vi "AAA Emrax 228 2.0 KLEIN BEELD.vi"() -> ()   [LabVIEW 2020]
doc: "This is a practical example of CAN_READ.\nOn the left hand side of the BD is a disabled code section. One can enable this to log CAN data.\nThe potput of this disabled code segment is the error cluster.\nThan the selected channel will be initiatlized.\nOnce the initialisation is OK a timed while loop will be executed until CAN_READ will signal an error.\nInside of the while loop is the CAN_READ function.\nBuilding up an array of CAN mesages and timestamps is done while this loop executes.\nOnly the last message witch is naturaly empty, because the receive queue is empty, will be ignored.\nThe result is an array of received CAN messages."
uses:
  <instrlib>/KDI Digital Instrumentation/API_for_PCAN_BASIC_FD/TPCANParameter.ctl
  <vilib>/Platform/TimedLoop/XDataNode/XDataNode.xnode
  <vilib>/Platform/TimedLoop/XDataNode/nitl_modes.ctl
  <vilib>/Platform/TimedLoop/XDataNode/XDNodeRunTimeDep.lvlib
  <vilib>/Platform/TimedLoop/XDataNode/wakeup.ctl
  <vilib>/Platform/TimedLoop/XDataNode/timing_clust.ctl
  <instrlib>/KDI Digital Instrumentation/API_for_PCAN_BASIC_FD/TPCANHandle.ctl
  <instrlib>/KDI Digital Instrumentation/API_for_PCAN_BASIC_FD/TPCANBaudrate.ctl
  <instrlib>/Gantner Instruments/Ethernet/Gantner-Instruments HighSpeedPort.llb/e.gate Protocol Type.ctl
  <vilib>/Instr/_visa.llb/VISA Configure Serial Port (Instr).vi
  <vilib>/Utility/file.llb/Write Delimited Spreadsheet (string).vi
  <instrlib>/KDI Digital Instrumentation/API_for_PCAN_BASIC_FD/PCAN Get CHANNEL CONDITION.vi
  <instrlib>/KDI Digital Instrumentation/API_for_PCAN_BASIC_FD/TPCANTimestampFD.ctl
panel:
  out "DC Current":dbl(knob) scale=0.0..140.0
  out "Array 2":u8[][](array[numeric])
  out "Max. Cell Voltage":dbl
  out "DC Voltage":dbl(knob) scale=80.0..120.0
  out "Array":u8[][](array[numeric])
  in  "?":bool
  out "error out 3":errorcluster
  out "error out":errorcluster
  out "Value":dbl[](graph)
  out "Brake pot Input":u32
  out "Torque Shudder":u32
  out "Motor Temp":u32(slide) scale=0.0..100.0
  out "Inverter Temp":u32(slide) scale=0.0..100.0
  out "Modulation":u32
  out "Motor Voltage Magnitude":u32
  out "Flux weakening regulator":u32
  out "RPM Feedback":u32(knob) scale=0.0..6000.0
  out "?":u32(knob) scale=0.0..60.0
  out "?":u32(knob) scale=0.0..60.0
  out "Torque Command":u32
  out "Torque Feedback":u32
  out "Potmeter Input":u32
  out "Elapsed Time":u32
  out "return count":u32
  out "Humidity (%)":string
  out "Pressure (Pa)":string
  out "Temperature (°C)":string
  out "Elapsed Time 2":string
  out "?":dbl[](array[slide]) scale=0.0..1000.0
  out "Temperature 2":dbl[](array[slide]) caption="Thermocouple 1" scale=20.0..50.0
  out "error out 2":errorcluster
  out "Min. Cell Voltage":dbl
  out "x/y":dbl(graph)
  out "Battery Temperature":u8(slide) scale=0.0..50.0
  out "State of Charge":dbl(slide) scale=0.0..100.0
  out "appended array":u8[][](array[numeric])
  out "CAN Timestamp":T1[](array[typedef]) format="%016x"
  # "Emrax 228  -  Motor control"
  # "Atmospheric\nConditions"
  # "Temperatures"
  # "Battery Data"
  # "Power Supply"
  # "Torque"
  # "DC Voltage"
  # "Thrust"
  # "DC Current"
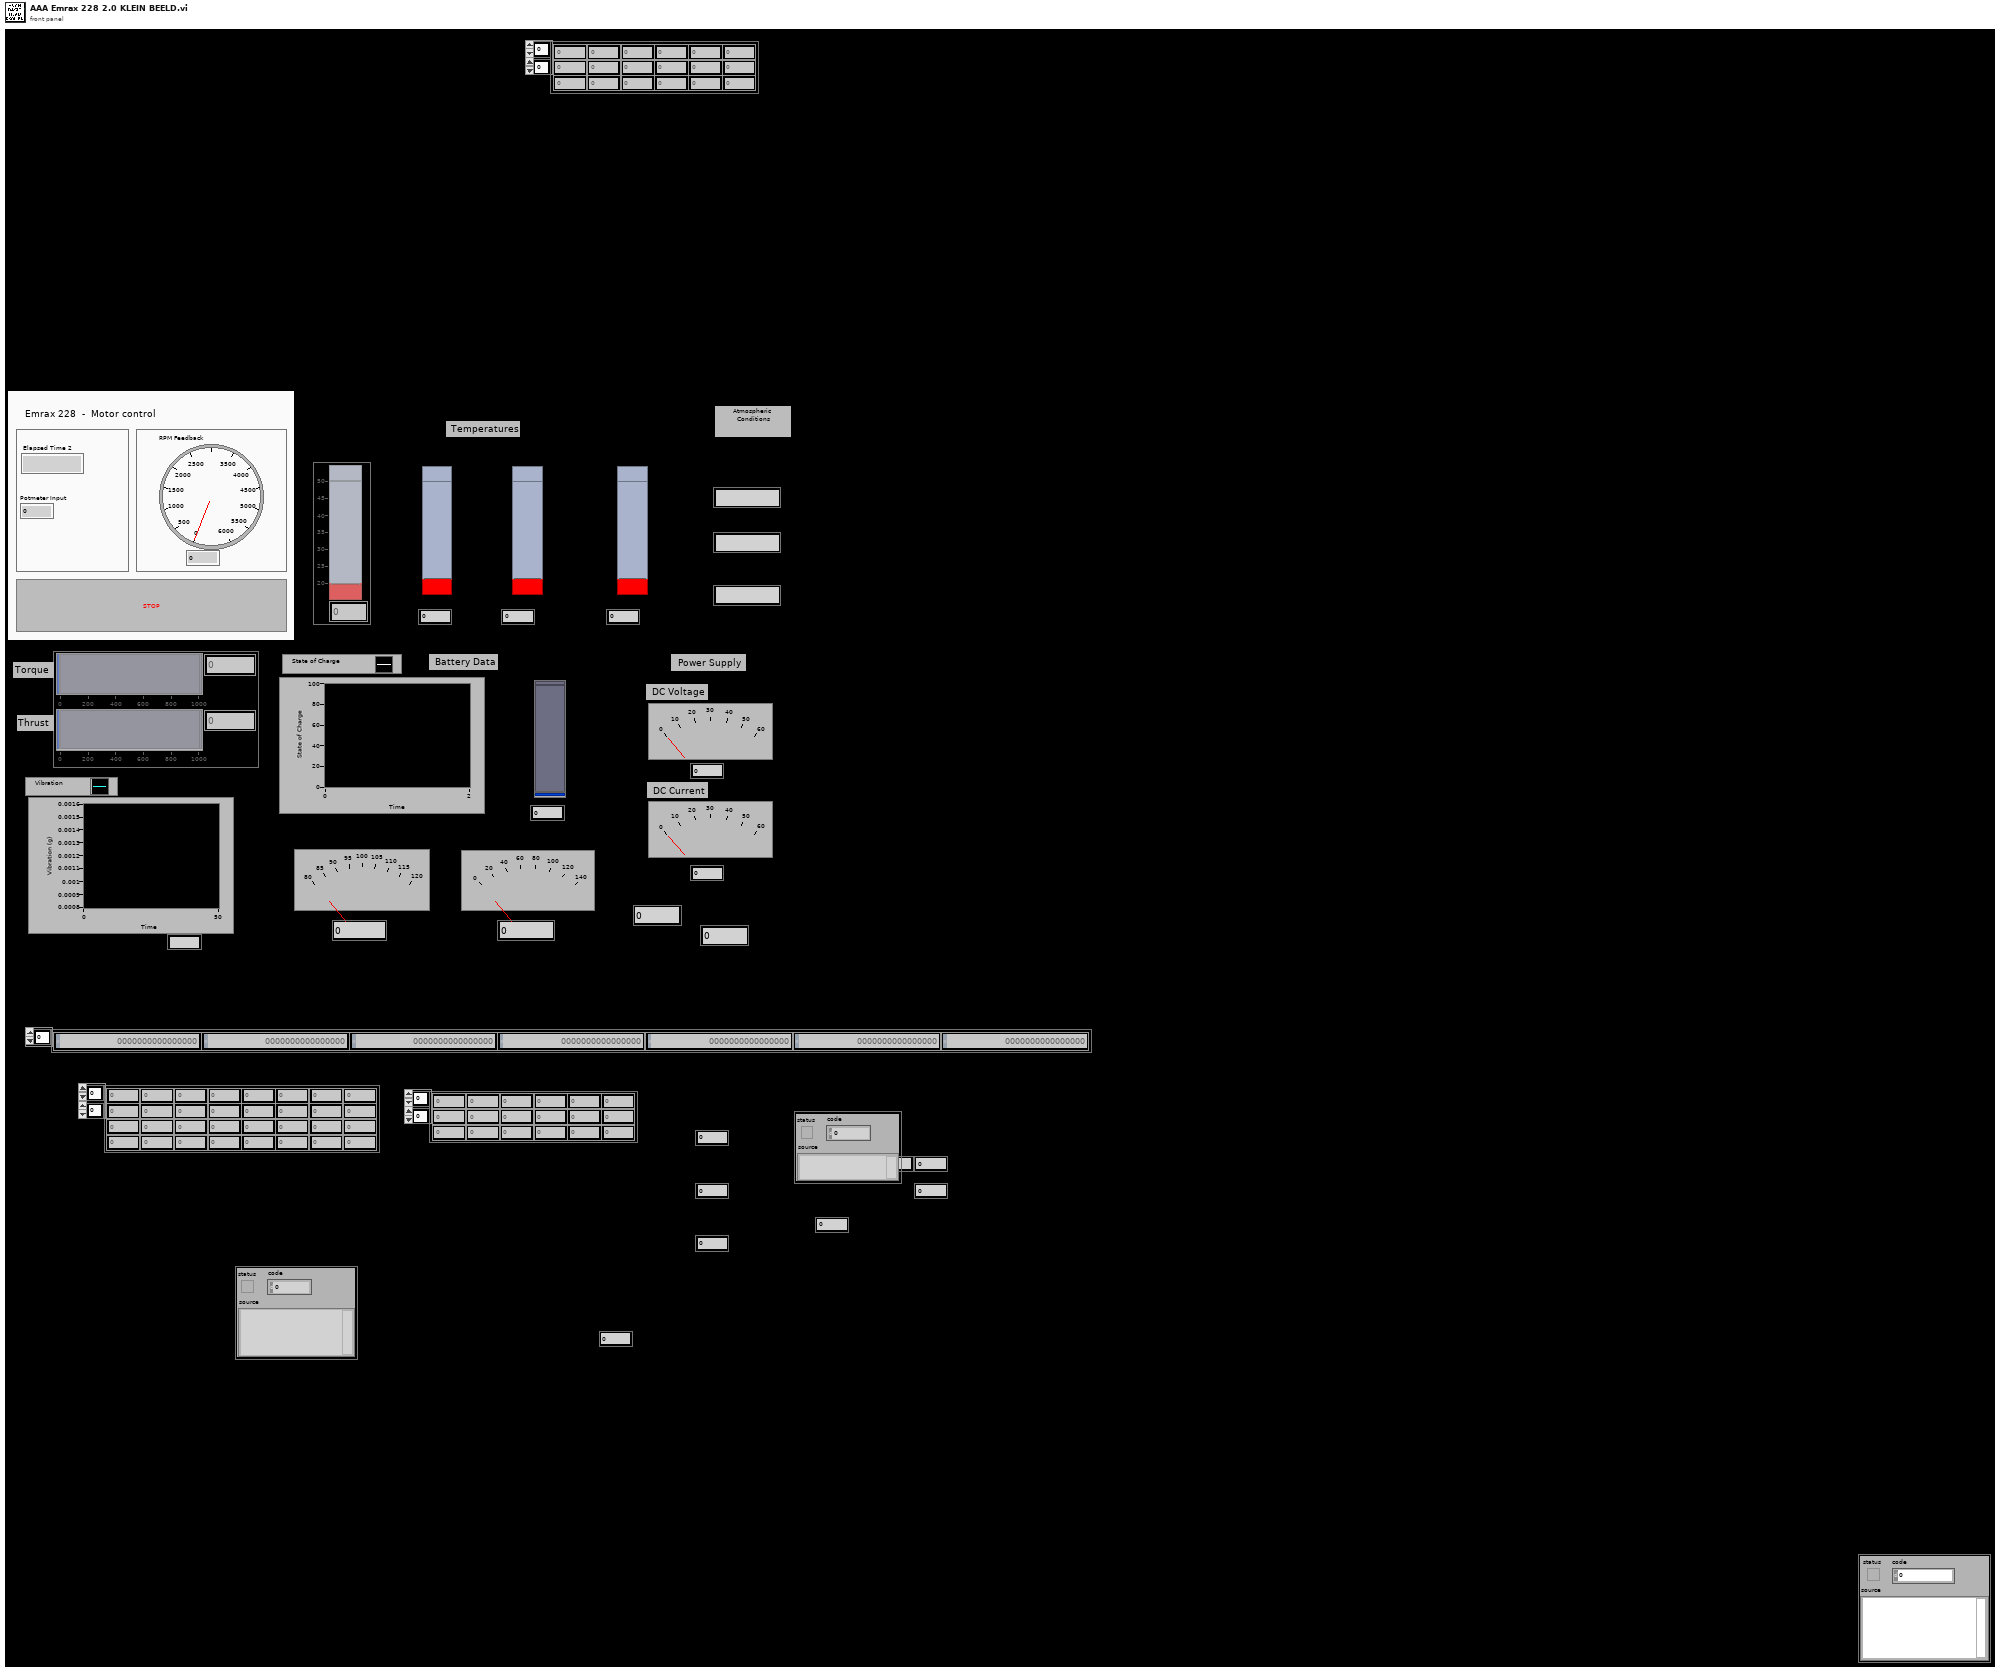
[diagram p1: front panel]
types:
  T1 = typedef "TPCANTimestampFD.ctl" = u64
  T2 = typedef "e.gate Protocol Type.ctl" = enum16{"ASCII", "HighspeedPort Online", "HighspeedPort Buffer (giutility.DLL) ", "PostProcessBuffer (giutility.DLL)", "HighspeedPort Online (giutility.DLL)", "Decode UDBF File (giutility.DLL)"}
  T3 = typedef "TPCANBaudrate.ctl" = enum16{"PCAN_BAUD_1M 0x0014", "PCAN_BAUD_800K 0x0016", "PCAN_BAUD_500K 0x001C", "PCAN_BAUD_250K 0x011C", "PCAN_BAUD_125K 0x031C", "PCAN_BAUD_100K 0x432F", "PCAN_BAUD_95K 0xC34E", "PCAN_BAUD_83K 0x852B", "PCAN_BAUD_50K 0x472F", "PCAN_BAUD_47K 0x1414", "PCAN_BAUD_33K 0x8B2F", "PCAN_BAUD_20K 0x532F", "PCAN_BAUD_10K 0x672F", "PCAN_BAUD_5K 0x7F7F", "User Baudrate"}
  T4 = typedef "TPCANHandle.ctl" = enum16{"PCAN_NONEBUS  0x000", "PCAN_ISABUS1  0x21", "PCAN_ISABUS2  0x22", "PCAN_ISABUS3  0x23", "PCAN_ISABUS4  0x24", "PCAN_ISABUS5  0x25", "PCAN_ISABUS6  0x26", "PCAN_ISABUS7  0x27", "PCAN_ISABUS8  0x28", "PCAN_DNGBUS1  0x31", "PCAN_PCIBUS1  0x41", "PCAN_PCIBUS1  0x42", "PCAN_PCIBUS1  0x43", "PCAN_PCIBUS1  0x44", "PCAN_PCIBUS1  0x45", "PCAN_PCIBUS1  0x46", "PCAN_PCIBUS1  0x47", "PCAN_PCIBUS1  0x48", "PCAN_PCIBUS1  0x409", "PCAN_PCIBUS1  0x40A", "PCAN_PCIBUS1  0x40B", "PCAN_PCIBUS1  0x40C", "PCAN_PCIBUS1  0x40D", "PCAN_PCIBUS1  0x40E", "PCAN_PCIBUS1  0x40F", "PCAN_PCIBUS1  0x410", "PCAN_USBBUS1  0x51", "PCAN_USBBUS2  0x52", "PCAN_USBBUS3  0x53", "PCAN_USBBUS4  0x54", "PCAN_USBBUS5  0x55", "PCAN_USBBUS6  0x56", "PCAN_USBBUS7  0x57", "PCAN_USBBUS8  0x58", "PCAN_USBBUS9  0x509", "PCAN_USBBUS10  0x50A", "PCAN_USBBUS11  0x50B", "PCAN_USBBUS12  0x50C", "PCAN_USBBUS13  0x50D", "PCAN_USBBUS14  0x50E", "PCAN_USBBUS15  0x50F", "PCAN_USBBUS16  0x510", "PCAN_PCCBUS1  0x61", "PCAN_PCCBUS2  0x62", "PCAN_LANBUS1  0x801", "PCAN_LANBUS2  0x802", "PCAN_LANBUS3  0x803", "PCAN_LANBUS4  0x804", "PCAN_LANBUS5  0x805", "PCAN_LANBUS6  0x806", "PCAN_LANBUS7  0x807", "PCAN_LANBUS8  0x808", "PCAN_LANBUS9  0x809", "PCAN_LANBUS10  0x80A", "PCAN_LANBUS11  0x80B", "PCAN_LANBUS12  0x80C", "PCAN_LANBUS13  0x80D", "PCAN_LANBUS14  0x80E", "PCAN_LANBUS15  0x80F", "PCAN_LANBUS16  0x810"}
  T5 = typedef "TPCANParameter.ctl" = enum8{"Not Available", "PCAN device number", "PCAN 5-volt power", "PCAN receive event", "PCAN message filter", "PCAN API version", "PCAN channel version", "PCAN busoff autoreset", "PCAN listen-only", "PCAN log location", "PCAN log status", "PCAN log configure", "PCAN log text", "PCAN channel condition", "PCAN hardware name", "PCAN_RECEIVE_STATUS", "PCAN_CONTROLLER_NUMBER", "PCAN_TRACE_LOCATION ", "PCAN_TRACE_STATUS", "PCAN_TRACE_SIZE", "PCAN_TRACE_CONFIGURE", "PCAN_CHANNEL_IDENTIFYING", "PCAN_CHANNEL_FEATURES", "PCAN_SPEED_ADAPTING", "PCAN_BITRATE_INFO", "PCAN_BITRATE_INFO_FD", "PCAN_BUSSPEED_NOMINAL", "PCAN_BUSSPEED_DATA", "PCAN_IP_ADDRESS", "PCAN_LAN_SERVICE_STATUS", "PCAN_ALLOW_STATUS_FRAMES", "PCAN_ALLOW_RTR_FRAMES", "PCAN_ALLOW_ERROR_FRAMES", "PCAN_INTERFRAME_DELAY", "PCAN_ACCEPTANCE_FILTER_11BIT", "PCAN_ACCEPTANCE_FILTER_29BIT", "PCAN_IO_DIGITAL_CONFIGURATION", "PCAN_IO_DIGITAL_VALUE", "PCAN_IO_DIGITAL_SET", "PCAN_IO_DIGITAL_CLEAR", "PCAN_IO_ANALOG_VALUE"}
  T6 = typedef "Channel Availability.ctl" = enum16{"PCAN_CHANNEL_UNAVAILABLE", "PCAN_CHANNEL_AVAILABLE", "PCAN_CHANNEL_OCCUPIED"}
  T7 = typedef "e.gate Configuration.ctl" = cluster{"connection ID":refnum<k5>, "IPAddress":string, "BufferIndex":i32, "StateMessage":string, "StateCode":i8, "HeaderSize":i32, "BufferSize":i32, "IsBigEndian":i32, "Version":i32, "ChannelCount":i32, "FrameLength":i32, "StartTime":dbl, "dActTimeToSecondFactor":dbl, "StartTimeToDayFactor":dbl, "BufferFillRate":dbl, "SampleRate":dbl, "ChannelData":T8[], "DecodeTimeFormat":string, "SummaryPath":string, "WithCheckSum":i32, "dActTimeDataType":T9, "MaxWriteCount":i32, "MaxReadCount":i32, "TempOffsetRead":i32, "TempLengthRead":i32, "Protocol":T2, "IsSupported":i32, "InputAccessList":i32[], "OutputAccessList":i32[], "DataSource":enum16{"CircleBuffer", "test.con Logger", "test.con Archive"}, "Modules":T10[], "DLL-Handle":T11}
  T8 = typedef "e.gate Channel Data.ctl" = cluster{"VariableName":string, "DataDirection":string, "DataType":string, "DataTypeIndex":T9, "Precision":i16, "FieldLengtht":i16, "ByteCount":i32, "Format":string, "Unit":string, "InputAccessOffset":i32, "OutputAccessOffset":i16, "InputAccessIndex":i16, "OutputAccessIndex":i16, "VarType":string}
  T9 = typedef "e.gate Data Type.ctl" = enum16{"NO", "BOOL", "SINT8", "USINT8", "SINT16", "USINT16", "SINT32", "USINT32", "FLOAT", "SET8", "SET16", "SET32", "DOUBLE", "SINT64", "USINT64", "SET64"}
  T10 = typedef "e.gate Module  Data.ctl" = cluster{"Type":string, "Location":string, "VariablesCount":i16, "UartIndex":i16, "Address":i16, "SystemOffset":i16}
  T11 = typedef "e.gateHSP_DLLhandle.ctl" = cluster{"clientInstance":i32, "connectionInstance":i32, "Is32Bit":bool, "DLL Path":path}
  T12 = typedef "XDNodeRunTimeDep.lvlib/timing_clust.ctl" = cluster{"Expected End [f-1]":u64, "Actual End [f-1]":u64, "Finished Late? [f-1]":bool, "Expected End [i-1]":u64, "Actual End [i-1]":u64, "Finished Late? [i-1]":bool, "Expected Start [i]":u64, "Actual Start [i]":u64, "Expected Start [f]":u64, "Actual Start [f]":u64, "Source Name":string, "Structure Name":string, "Period":i64, "Deadline":i64, "Offset":i64, "Start":i64, "Priority":i32, "Timeout":i32, "Mode":T13, "Wakeup Reason":T14, "Error":errorcluster, "Source Type":string, "Secondary Source Type":string, "Global End Time":u64, "Global Start Time":u64, "Frame Duration":u64, "Iteration Duration":u64, "Assigned CPU":i32, "I/O Scan Engine Mode":u32}
  T13 = typedef "XDNodeRunTimeDep.lvlib/nitl_modes.ctl" = enum32{"No Change", "Process missed periods, maintain original phase", "Discard missed periods, maintain original phase", "Process missed periods, ignore original phase", "Discard missed periods, ignore original phase"}
  T14 = typedef "XDNodeRunTimeDep.lvlib/wakeup.ctl" = enum32{"Normal", "Aborted", "Asynchronous wakeup", "Timing source error", "Timed loop error", "Timeout"}
  T15 = typedef "CAN MSG Cluster.ctl" = cluster{"ID":u32, "MSG type":u8, "DLC":u8, "DATA":u8[]}
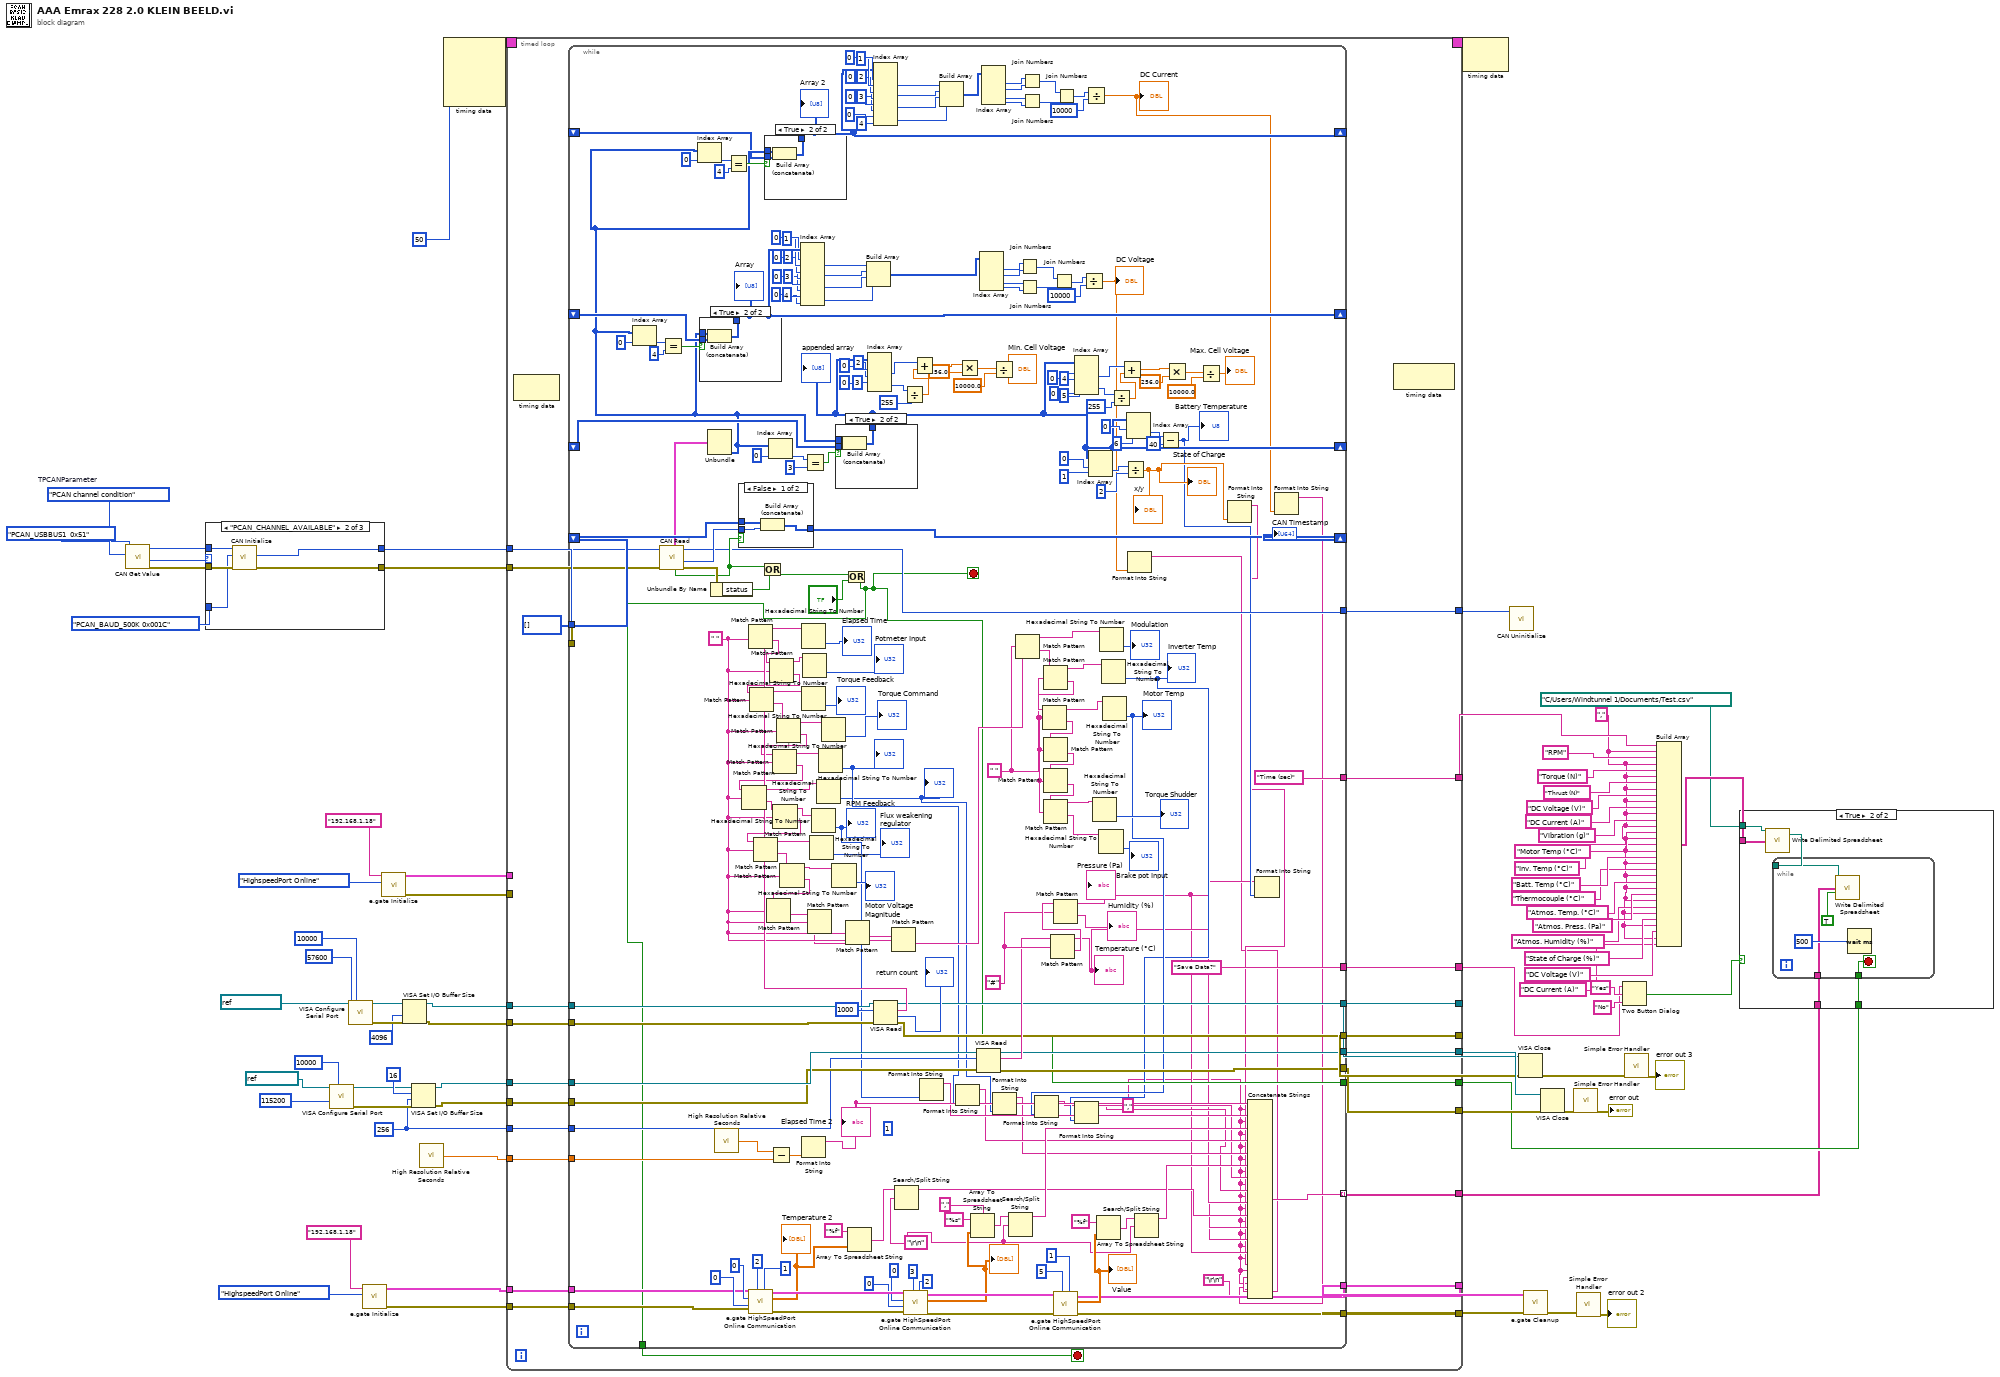
[diagram p0: block diagram]
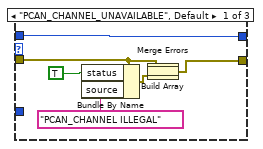
[diagram p7: hidden frame]
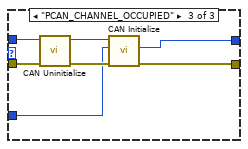
[diagram p8: hidden frame]
diagram:
  w2 = "," ("element")
  w42 = u32 256 ("buffer size")
  w76 = TPCANParameter."PCAN channel condition"  # TPCANParameter
  n1 = call-poly <instrlib>:"CAN Get Value.vi"("TPCANParameter"=w76, "TPCANHandle"=TPCANHandle."PCAN_USBBUS1  0x51") -> ("error out"=w73:errorcluster, "Channel condition"=w72:T6, "TPCANHandle out"=w74:T4)  [unwired: 7 in]
  n2 = case shown="\"PCAN_CHANNEL_AVAILABLE\"" w72 {
    tunnel: [w82 w88 w92] -> w69
    tunnel: w74 -> [w83 w87 w94]
    tunnel: w73 -> [w81 w86 w95]
    tunnel: TPCANBaudrate."PCAN_BAUD_500K 0x001C" ("TPCANBaudrate") -> [_ w84 w89]
    tunnel: [w83 w85 w90] -> w70
    frame "PCAN_CHANNEL_UNAVAILABLE", Default {
      n3 = Bundle By Name(cluster=w81, "status"=TRUE, "source"="PCAN_CHANNEL ILLEGAL") -> (w78:errorcluster)
      n4 = Build Array(w81, w78) -> (w77:errorcluster[])
      n5 = Merge Errors(w77) -> (w82:errorcluster)
    }
    frame "PCAN_CHANNEL_AVAILABLE" {
      n6 = call <instrlib>:"CAN Initialize.vi"("error in (no error)"=w86, "TPCANBaudrate"=w84, "TPCANHandle"=w87) -> ("error out"=w88:errorcluster, "TPCANHandle_out"=w85:T4)  [unwired: 6 in, 1 out]
    }
    frame "PCAN_CHANNEL_OCCUPIED" {
      n7 = call <instrlib>:"CAN Uninitialize.vi"("error in (no error)"=w95, "TPCANHandle"=w94) -> ("error out"=w93:errorcluster, "TPCANHandle out"=w91:T4)  [unwired: 7 in, 1 out]
      n8 = call <instrlib>:"CAN Initialize.vi"("error in (no error)"=w93, "TPCANBaudrate"=w89, "TPCANHandle"=w91) -> ("error out"=w92:errorcluster, "TPCANHandle_out"=w90:T4)  [unwired: 6 in, 1 out]
    }
  }
  n9 = call-poly "VISA Configure Serial Port"("VISA resource name"=refnum<visa-resource-name> "COM5", "timeout (10sec)"=u32 10000, "baud rate (9600)"=u32 115200) -> ("VISA resource name out"=w59:refnum<visa-resource-name>, "error out"=w58:errorcluster)  [unwired: 11 in]
  n10 = call-poly "VISA Configure Serial Port"("VISA resource name"=refnum<visa-resource-name> "COM6", "timeout (10sec)"=u32 10000, "baud rate (9600)"=u32 57600) -> ("VISA resource name out"=w52:refnum<visa-resource-name>, "error out"=w51:errorcluster)  [unwired: 11 in]
  n11 = call <instrlib>:"e.gate Initialize.vi"("Protocol"=e.gate_Protocol_Type."HighspeedPort Online", "IP Address"="192.168.1.18") -> ("error out"=w39:errorcluster, "e.gate Configuration"=w40:T7)  [unwired: 8 in]
  n12 = call <instrlib>:"e.gate Initialize.vi"("Protocol"=e.gate_Protocol_Type."HighspeedPort Online", "IP Address"="192.168.1.18") -> ("error out"=w61:errorcluster, "e.gate Configuration"=w62:T7)  [unwired: 8 in]
  n13 = VISA Set I/O Buffer Size(VISA resource name=w52, size (4096)=u32 4096, error in (no error)=w51) -> (VISA resource name out=w46:refnum<visa-resource-name>, error out=w45:errorcluster)  [unwired: 1 in]
  n14 = VISA Set I/O Buffer Size(VISA resource name=w59, mask (16)=u16 16 ("I/O Receive\nBuffer mask"), size (4096)=w42, error in (no error)=w58) -> (VISA resource name out=w44:refnum<visa-resource-name>, error out=w43:errorcluster)
  n15 = call <vilib>:"High Resolution Relative Seconds.vi"() -> ("relative seconds"=w41:dbl)
  n16 = node-c288(i64 50 ("Period")) -> (w68:T12)  [unwired: 3 in]
  n17 = timed-loop {
    timing: w68 -> [_]
    timing-out: [_] -> w67
    tunnel: w70 -> [w119]
    tunnel: w69 -> [w118]
    tunnel: [w116] -> w38
    tunnel: w62 -> [_]
    tunnel: w61 -> [_]
    tunnel: w46 -> [w115]
    tunnel: w45 -> [w114]
    tunnel: w44 -> [w113]
    tunnel: w43 -> [w112]
    tunnel: w42 -> [w111]
    tunnel: w41 -> [w110]
    tunnel: w40 -> [w109]
    tunnel: w39 -> [w108]
    tunnel: [w106] -> w37
    tunnel: [w105] -> w36
    tunnel: [w104] -> w25
    tunnel: [w103] -> w24
    tunnel: [w102] -> w23
    tunnel: [w101] -> w22
    tunnel: [w100] -> w21
    tunnel: [w99] -> w20
    tunnel: [w97] -> w19
    tunnel: [w96] -> w7
    stop <- w98 stop-if-true
    n18 = node-c288() -> ()  [unwired: 1 in, 1 out]
    n19 = while {
      tunnel: w119 -> [w347]
      tunnel: w118 -> [w346]
      tunnel: [w176] -> w98
      shift-right: [w342] -> w107
      shift-left: u64[] [] -> [w343]
      tunnel: [w340] -> w116
      shift-right: [w190] -> _
      shift-left: _ -> [w328]
      tunnel: w115 -> [w234]
      tunnel: w114 -> [w233]
      tunnel: w113 -> [w232]
      tunnel: w112 -> [w231]
      tunnel: w111 -> [w230]
      tunnel: w110 -> [w229]
      tunnel: w109 -> [w228]
      tunnel: w108 -> [w227]
      tunnel: [w226] -> w106
      tunnel: [w225] -> w105
      tunnel: [w224] -> w104
      tunnel: [w223] -> w103
      tunnel: [w176] -> w102
      tunnel: ["Save Data?" ("message")] -> w101
      tunnel: [w221] -> w100
      tunnel: [w220] -> w99
      shift-right: [w212] -> _
      shift-left: _ -> [w213]
      tunnel: ["Time (sec)" ("element")] -> w97
      tunnel: [w165] -> w96 mode=indexing
      shift-right: [w125] -> _
      shift-left: _ -> [w124]
      stop <- w176 stop-if-true
      w235 = "\r\n" ("search string/char (-)")
      w257 = " " ("search string/char (-)")
      w267 = " " ("search string/char (-)")
      w293 = "#" ("regular expression")
      (unwired) 1 ("offset (0)")
      w122 = "," ("string")
      n20 = call <instrlib>:"CAN Read.vi"("error in (no error)"=w346, "TPCANHandle"=w347) -> ("error out"=w345:errorcluster, "TPCANTimestamp out"=w341:T1, "CAN_Message out"=w339:T15, "TPCANHandle out"=w340:T4, "rcv queue empty"=w344:bool)  [unwired: 5 in]
      n21 = Unbundle(w339) -> ("DATA"=w126:u8[])  [unwired: 3 out]
      n22 = Index Array(array=w126, index=0) -> (element=w216:u8)
      n23 = Equal?(x=w216, y=u8 4) -> (x = y?=w214:bool)
      n24 = Index Array(array=w126, index=0) -> (element=w150:u8)
      n25 = case shown="True" w214 {
        tunnel: w126 -> [_ w355]
        tunnel: w213 -> [w352 w354]
        tunnel: [w352 w353] -> w212
        frame False {
        }
        frame True {
          n26 = Build Array (concatenate)(w355, w354) -> (w353:u8[][])
        }
      }
      "Array" <- w212
      n27 = Unbundle By Name(w345) -> ("status"=w312:bool)
      n28 = call <vilib>:"High Resolution Relative Seconds.vi"() -> ("relative seconds"=w300:dbl)
      n29 = Equal?(x=w150, y=u8 4) -> (x = y?=w148:bool)
      n30 = case shown="False" w344 {
        tunnel: w343 -> [w362 w363]
        tunnel: w341 -> [w361 _]
        tunnel: [w360 w363] -> w342
        frame False {
          n31 = Build Array (concatenate)(w362, w361) -> (w360:T1[])
        }
        frame True {
        }
      }
      n32 = call <instrlib>:"e.gate HighSpeedPort Online Communication.vi"("ReadCount"=1, "ReadIndex"=2, "error in (no error)"=w227, "WriteCount"=0, "WriteIndex"=0, "e.gate Configuration In"=w228) -> ("error out"=w306:errorcluster, "Value"=w301:dbl[], "e.gate Configuration Out"=w307:T7)  [unwired: 3 in]
      "Temperature 2" <- w301
      n33 = Or(x=w344, y=w312) -> (x .or. y?=w219:bool)
      n34 = case shown="True" w148 {
        tunnel: w126 -> [_ w351]
        tunnel: w124 -> [w348 w350]
        tunnel: [w348 w349] -> w125
        frame False {
        }
        frame True {
          n35 = Build Array (concatenate)(w351, w350) -> (w349:u8[][])
        }
      }
      "Array 2" <- w125
      n36 = Index Array(array=w126, index=0) -> (element=w330:u8)
      n37 = Subtract(x=w300, y=w229) -> (x-y=w299:dbl)
      n38 = Index Array(array=w212, index (row) #1=0 ("index (row)"), index (col) #1=1 ("disabled index (col)"), index (row) #2=0 ("index (row)"), index (col) #2=2 ("disabled index (col)"), index (row) #3=0 ("index (row)"), index (col) #3=3 ("disabled index (col)"), index (row) #4=0 ("index (row)"), index (col) #4=4 ("disabled index (col)")) -> (element #1=w203:u8, element #2=w202:u8, element #3=w201:u8, element #4=w200:u8)
      n39 = Format Into String(w299) -> (resulting string=w174:string)  [unwired: 3 in, 1 out]
      "Elapsed Time 2" <- w174
      n40 = Equal?(x=w330, y=u8 3) -> (x = y?=w327:bool)
      n41 = case shown="True" w327 {
        tunnel: w126 -> [_ w359]
        tunnel: w328 -> [w356 w358]
        tunnel: [w356 w357] -> w190
        frame False {
        }
        frame True {
          n42 = Build Array (concatenate)(w359, w358) -> (w357:u8[][])
        }
      }
      "appended array" <- w190
      n43 = Or(x=w219, y="?") -> (x .or. y?=w176:bool)
      n44 = Array To Spreadsheet String(array=w301, 3:"%f" ("format string")) -> (spreadsheet string=w295:string)  [unwired: 1 in]
      n45 = Build Array(w203, w202, w201, w200) -> (w199:u8[])
      n46 = Index Array(array=w190, index (row) #1=0 ("index (row)"), index (col) #1=2 ("disabled index (col)"), index (row) #2=0 ("index (row)"), index (col) #2=3 ("disabled index (col)")) -> (element #1=w324:u8, element #2=w321:u8)
      n47 = Index Array(array=w125, index (row) #1=0 ("index (row)"), index (col) #1=1 ("disabled index (col)"), index (row) #2=0 ("index (row)"), index (col) #2=2 ("disabled index (col)"), index (row) #3=0 ("index (row)"), index (col) #3=3 ("disabled index (col)"), index (row) #4=0 ("index (row)"), index (col) #4=4 ("disabled index (col)")) -> (element #1=w140:u8, element #2=w139:u8, element #3=w138:u8, element #4=w127:u8)
      n48 = VISA Read(VISA resource name=w234, byte count=u32 1000, error in (no error)=w233) -> (VISA resource name out=w221:refnum<visa-resource-name>, read buffer=w284:string, return count=→"return count":u32, error out=w220:errorcluster)
      n49 = Match Pattern(string=w284, regular expression=w267) -> (before substring=w271:string, after substring=w273:string)  [unwired: 1 in, 2 out]
      n50 = Match Pattern(string=w273, regular expression=w267) -> (before substring=w274:string, after substring=w276:string)  [unwired: 1 in, 2 out]
      n51 = Match Pattern(string=w276, regular expression=w267) -> (before substring=w277:string, after substring=w279:string)  [unwired: 1 in, 2 out]
      n52 = Match Pattern(string=w279, regular expression=w267) -> (before substring=w280:string, after substring=w282:string)  [unwired: 1 in, 2 out]
      n53 = Match Pattern(string=w282, regular expression=w267) -> (before substring=w240:string, after substring=w283:string)  [unwired: 1 in, 2 out]
      n54 = Match Pattern(string=w283, regular expression=w267) -> (before substring=w239:string, after substring=w285:string)  [unwired: 1 in, 2 out]
      n55 = Match Pattern(string=w285, regular expression=w267) -> (before substring=w243:string, after substring=w286:string)  [unwired: 1 in, 2 out]
      n56 = Match Pattern(string=w286, regular expression=w267) -> (before substring=w287:string, after substring=w289:string)  [unwired: 1 in, 2 out]
      n57 = Match Pattern(string=w289, regular expression=w267) -> (before substring=w290:string, after substring=w268:string)  [unwired: 1 in, 2 out]
      n58 = Match Pattern(string=w268, regular expression=w267) -> (after substring=w266:string)  [unwired: 1 in, 3 out]
      n59 = Hexadecimal String To Number(string=w271) -> (number=→"Elapsed Time":u32)  [unwired: 2 in, 1 out]
      n60 = Hexadecimal String To Number(string=w277) -> (number=→"Torque Feedback":u32)  [unwired: 2 in, 1 out]
      n61 = Hexadecimal String To Number(string=w274) -> (number=→"Potmeter Input":u32)  [unwired: 2 in, 1 out]
      n62 = Match Pattern(string=w266, regular expression=w267) -> (after substring=w265:string)  [unwired: 1 in, 3 out]
      n63 = Hexadecimal String To Number(string=w287) -> (number=→"Flux weakening regulator":u32)  [unwired: 2 in, 1 out]
      n64 = Hexadecimal String To Number(string=w243) -> (number=w173:u32)  [unwired: 2 in, 1 out]
      "RPM Feedback" <- w173
      n65 = Hexadecimal String To Number(string=w239) -> (number=w152:u32)  [unwired: 2 in, 1 out]
      "?" <- w152
      n66 = Hexadecimal String To Number(string=w240) -> (number=w169:u32)  [unwired: 2 in, 1 out]
      "?" <- w169
      n67 = Hexadecimal String To Number(string=w280) -> (number=→"Torque Command":u32)  [unwired: 2 in, 1 out]
      n68 = Hexadecimal String To Number(string=w290) -> (number=→"Motor Voltage Magnitude":u32)  [unwired: 2 in, 1 out]
      n69 = Match Pattern(string=w265, regular expression=w267) -> (after substring=w264:string)  [unwired: 1 in, 3 out]
      n70 = Match Pattern(string=w264, regular expression=w267) -> (after substring=w263:string)  [unwired: 1 in, 3 out]
      n71 = Search/Split String(string=w295, search string/char (-)=w235) -> (substring before match=w158:string)  [unwired: 1 in, 2 out]
      n72 = Divide(x=w321, y=u8 255) -> (x/y=w319:dbl)
      n73 = call <instrlib>:"e.gate HighSpeedPort Online Communication.vi"("ReadCount"=2, "ReadIndex"=3, "error in (no error)"=w306, "WriteCount"=0, "WriteIndex"=0, "e.gate Configuration In"=w307) -> ("error out"=w247:errorcluster, "Value"=w244:dbl[], "e.gate Configuration Out"=w248:T7)  [unwired: 3 in]
      "?" <- w244
      n74 = Add(x=w324, y=w319) -> (x+y=w318:dbl)
      n75 = Format Into String(w173) -> (resulting string=w172:string)  [unwired: 3 in, 1 out]
      n76 = Build Array(w140, w139, w138, w127) -> (w129:u8[])
      n77 = Format Into String(w169) -> (resulting string=w164:string)  [unwired: 3 in, 1 out]
      n78 = Multiply(x=w318, y=256.0) -> (x*y=w316:dbl)
      n79 = Array To Spreadsheet String(delimiter (Tab)=",", array=w244, 3:"%s" ("format string")) -> (spreadsheet string=w238:string)
      n80 = VISA Read(VISA resource name=w232, byte count=w230, error in (no error)=w231) -> (VISA resource name out=w224:refnum<visa-resource-name>, read buffer=w292:string, error out=w223:errorcluster)  [unwired: 1 out]
      n81 = Index Array(array=w199) -> (element #1=w197:u8, element #2=w198:u8, element #3=w196:u8, element #4=w195:u8)  [unwired: 4 in]
      n82 = Index Array(array=w129) -> (element #1=w136:u8, element #2=w137:u8, element #3=w135:u8, element #4=w134:u8)  [unwired: 4 in]
      n83 = Divide(x=w316, y=10000.0) -> (x/y=→"Min. Cell Voltage":dbl)
      n84 = Format Into String(w152) -> (resulting string=w163:string)  [unwired: 3 in, 1 out]
      n85 = Search/Split String(string=w238, search string/char (-)=w235) -> (substring before match=w171:string)  [unwired: 1 in, 2 out]
      n86 = Match Pattern(string=w263, regular expression=w257) -> (before substring=w256:string, after substring=w262:string)  [unwired: 1 in, 2 out]
      n87 = Join Numbers(hi=w197, lo=w198) -> ((hi.lo)=w193:u16)
      n88 = Join Numbers(hi=w196, lo=w195) -> ((hi.lo)=w194:u16)
      n89 = Join Numbers(hi=w136, lo=w137) -> ((hi.lo)=w132:u16)
      n90 = Join Numbers(hi=w135, lo=w134) -> ((hi.lo)=w133:u16)
      n91 = Match Pattern(string=w262, regular expression=w257) -> (before substring=w255:string, after substring=w261:string)  [unwired: 1 in, 2 out]
      n92 = Match Pattern(string=w261, regular expression=w257) -> (before substring=w254:string, after substring=w260:string)  [unwired: 1 in, 2 out]
      n93 = Match Pattern(string=w260, regular expression=w257) -> (after substring=w259:string)  [unwired: 1 in, 3 out]
      n94 = Match Pattern(string=w259, regular expression=w257) -> (after substring=w258:string)  [unwired: 1 in, 3 out]
      n95 = Match Pattern(string=w258, regular expression=w257) -> (before substring=w253:string, after substring=w249:string)  [unwired: 1 in, 2 out]
      n96 = Match Pattern(string=w292, regular expression=w293) -> (before substring=w157:string, after substring=w294:string)  [unwired: 1 in, 2 out]
      "Temperature (°C)" <- w157
      n97 = Join Numbers(hi=w193, lo=w194) -> ((hi.lo)=w192:u32)
      n98 = call <instrlib>:"e.gate HighSpeedPort Online Communication.vi"("ReadCount"=1, "ReadIndex"=5, "error in (no error)"=w247, "e.gate Configuration In"=w248) -> ("error out"=w225:errorcluster, "Value"=w242:dbl[], "e.gate Configuration Out"=w226:T7)  [unwired: 5 in]
      "Value" <- w242
      n99 = Match Pattern(string=w294, regular expression=w293) -> (before substring=w156:string, after substring=→"Humidity (%)":string)  [unwired: 1 in, 2 out]
      "Pressure (Pa)" <- w156
      n100 = Join Numbers(hi=w132, lo=w133) -> ((hi.lo)=w131:u32)
      n101 = Index Array(array=w190, index (row) #1=0 ("index (row)"), index (col) #1=4 ("disabled index (col)"), index (row) #2=0 ("index (row)"), index (col) #2=5 ("disabled index (col)")) -> (element #1=w177:u8, element #2=w178:u8)
      n102 = Divide(x=w192, y=u32 10000) -> (x/y=w154:dbl)
      "DC Voltage" <- w154
      n103 = Divide(x=w131, y=u32 10000) -> (x/y=w123:dbl)
      "DC Current" <- w123
      n104 = Index Array(array=w190, index (row)=0, index (col)=1 ("disabled index (col)")) -> (element=w337:u8)
      n105 = Hexadecimal String To Number(string=w253) -> (number=→"Torque Shudder":u32)  [unwired: 2 in, 1 out]
      n106 = Array To Spreadsheet String(array=w242, 3:"%f" ("format string")) -> (spreadsheet string=w236:string)  [unwired: 1 in]
      n107 = Hexadecimal String To Number(string=w249) -> (number=→"Brake pot Input":u32)  [unwired: 2 in, 1 out]
      n108 = Hexadecimal String To Number(string=w256) -> (number=→"Modulation":u32)  [unwired: 2 in, 1 out]
      n109 = Hexadecimal String To Number(string=w255) -> (number=w167:u32)  [unwired: 2 in, 1 out]
      "Inverter Temp" <- w167
      n110 = Format Into String(w167) -> (resulting string=w160:string)  [unwired: 3 in, 1 out]
      n111 = Hexadecimal String To Number(string=w254) -> (number=w168:u32)  [unwired: 2 in, 1 out]
      "Motor Temp" <- w168
      n112 = Format Into String(w168) -> (resulting string=w161:string)  [unwired: 3 in, 1 out]
      n113 = Divide(x=w178, y=u8 255) -> (x/y=w185:dbl)
      n114 = Add(x=w177, y=w185) -> (x+y=w184:dbl)
      n115 = Divide(x=w337, y=u8 2) -> (x/y=w175:dbl)
      "State of Charge" <- w175
      "x/y" <- w175
      n116 = Index Array(array=w190, index (row)=0, index (col)=6 ("disabled index (col)")) -> (element=w333:u8)
      n117 = Format Into String(w154) -> (resulting string=w153:string)  [unwired: 3 in, 1 out]
      n118 = Search/Split String(string=w236, search string/char (-)=w235) -> (substring before match=w162:string)  [unwired: 1 in, 2 out]
      n119 = Subtract(x=w333, y=u8 40) -> (x-y=w166:u8)
      "Battery Temperature" <- w166
      n120 = Multiply(x=w184, y=256.0) -> (x*y=w182:dbl)
      n121 = Divide(x=w182, y=10000.0) -> (x/y=→"Max. Cell Voltage":dbl)
      n122 = Format Into String(w175) -> (resulting string=w155:string)  [unwired: 3 in, 1 out]
      n123 = Format Into String(w166) -> (resulting string=w159:string)  [unwired: 3 in, 1 out]
      n124 = Format Into String(w123) -> (resulting string=w121:string)  [unwired: 3 in, 1 out]
      n125 = Concatenate Strings(w174, w122, w172, w122, w171, w122, w164, w122, w163, w122, w162, w122, w161, w122, w160, w122, w159, w122, w158, w122, w157, w122, w156, w122, w156, w122, w155, w122, w153, w122, w121, "\r\n") -> (w165:string)
    }
    "CAN Timestamp" <- w107
    n126 = node-c288() -> ()  [unwired: 1 in, 1 out]
  }
  n127 = node-c288(w67) -> ()  [unwired: 1 out]
  n128 = call <instrlib>:"CAN Uninitialize.vi"("TPCANHandle"=w38) -> ()  [unwired: 8 in, 3 out]
  n129 = VISA Close(VISA resource name=w21, error in (no error)=w20) -> (error out=w27:errorcluster)
  n130 = call <instrlib>:"e.gate Cleanup.vi"("error in (no error)"=w36, "e.gate Configuration"=w37) -> ("error out"=w66:errorcluster)  [unwired: 9 in]
  n131 = VISA Close(VISA resource name=w25, error in (no error)=w24) -> (error out=w35:errorcluster)
  n132 = call <vilib>:"Simple Error Handler.vi"("error in (no error)"=w35) -> ("error out"=→"error out":errorcluster)  [unwired: 4 in, 4 out]
  n133 = call <vilib>:"Simple Error Handler.vi"("error in (no error)"=w66) -> ("error out"=→"error out 2":errorcluster)  [unwired: 4 in, 4 out]
  n134 = Two Button Dialog(message=w22, 1:"No" ("F button name (\"Cancel\")"), 2:"Yes" ("T button name (\"OK\")")) -> (T button?=w32:bool)
  n135 = call <vilib>:"Simple Error Handler.vi"("error in (no error)"=w27) -> ("error out"=→"error out 3":errorcluster)  [unwired: 4 in, 4 out]
  n136 = Build Array(w19, w2, "RPM" ("element"), w2, "Torque (N)" ("element"), w2, "Thrust (N)" ("element"), w2, "DC Voltage (V)" ("element"), w2, "DC Current (A)" ("element"), w2, "Vibration (g)" ("element"), w2, "Motor Temp (°C)" ("element"), w2, "Inv. Temp (°C)" ("element"), w2, "Batt. Temp (°C)" ("element"), w2, "Thermocouple (°C)" ("element"), w2, "Atmos. Temp. (°C)" ("element"), w2, "Atmos. Press. (Pa)" ("element"), w2, "Atmos. Humidity (%)" ("element"), w2, "State of Charge (%)" ("element"), w2, "DC Voltage (V)" ("element"), w2, "DC Current (A)" ("element")) -> (w33:string[])
  n137 = case shown="True" w32 {
    tunnel: w33 -> [_ w369]
    tunnel: w23 -> [_ w368]
    tunnel: path "C:/Users/Windtunnel 1/Documents/Test.csv" ("file path (dialog if empty) 2") -> [_ w367]
    tunnel: w7 -> [_ w366]
    frame False {
    }
    frame True {
      n138 = call-poly <vilib>:"Write Delimited Spreadsheet.vi"("file path (dialog if empty)"=w367, "1D data"=w369) -> ("new file path (Not A Path if cancelled)"=w370:path)  [unwired: 12 in, 1 out]
      n139 = while {
        tunnel: w370 -> [w375]
        tunnel: w368 -> [w372]
        tunnel: w366 -> [w371]
        stop <- w372 stop-if-true
        n140 = call-poly <vilib>:"Write Delimited Spreadsheet.vi"("file path (dialog if empty)"=w375, "1D data"=w371, "append to file? (new file:F)"=TRUE) -> ()  [unwired: 11 in, 2 out]
        n141 = Wait (ms)(milliseconds to wait=u32 500) -> ()  [unwired: 1 out]
      }
    }
  }
